vi "PM-A-Acquisition_main_DAQmx.vi"(8 "error in":errorcluster, 11 "init_cluster":T1) -> (0 "error out":errorcluster)   [LabVIEW 2018]
uses:
  init-close/PM-init-data_cluster.ctl
  init-close/PM-init-user_events.ctl
  init-close/PM-common-heartrate_data.ctl
  init-close/PM-common-peak-detect_settings.ctl
  PM-A-aqn_loop_data.ctl
panel:
  in  "Stop":bool
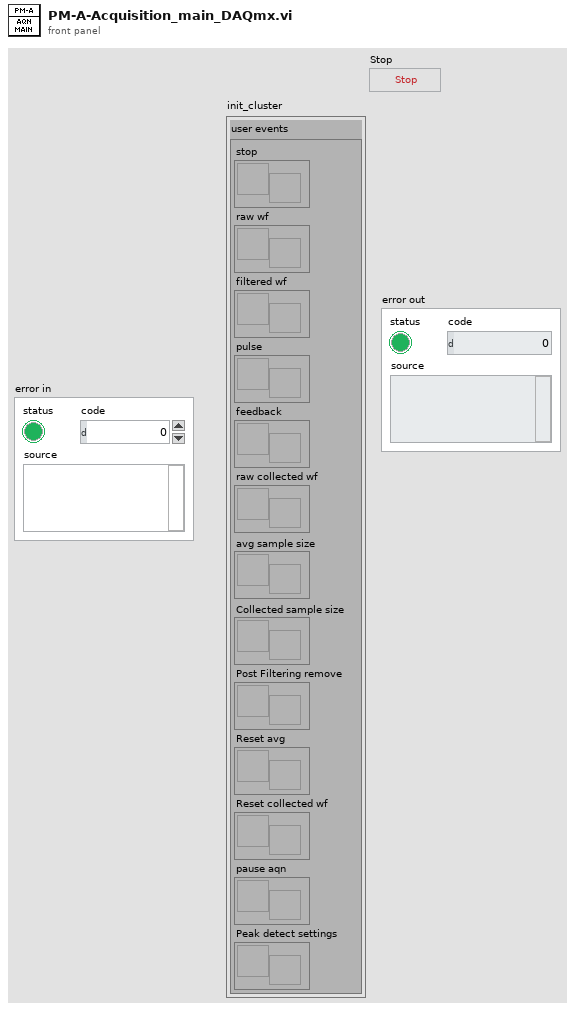
[diagram p1: front panel]
types:
  T1 = typedef "PM-init-data_cluster.ctl" = cluster{"user events":T2}
  T2 = typedef "PM-init-user_events.ctl" = cluster{"stop":refnum<user-event>, "raw wf":refnum<user-event>, "filtered wf":refnum<user-event>, "pulse":refnum<user-event>, "feedback":refnum<user-event>, "raw collected wf":refnum<user-event>, "avg sample size":refnum<user-event>, "Collected sample size":refnum<user-event>, "Post Filtering remove":refnum<user-event>, "Reset avg":refnum<user-event>, "Reset collected wf":refnum<user-event>, "pause aqn":refnum<user-event>, "Peak detect settings":refnum<user-event>}
  T3 = typedef "PM-A-aqn_loop_data.ctl" = cluster{"Stop event":refnum<user-event>, "Raw wf event":refnum<user-event>}
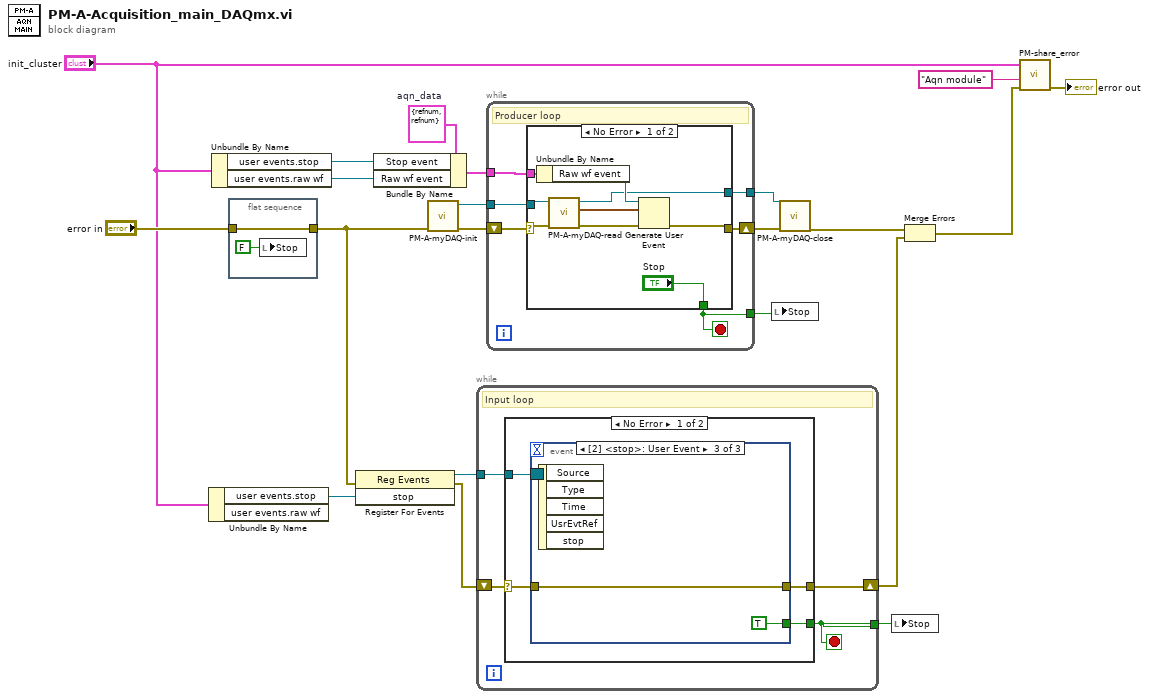
[diagram p0: block diagram]
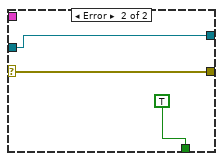
[diagram p2: hidden frame]
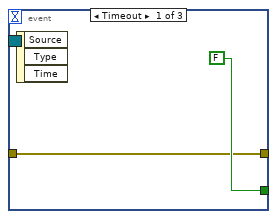
[diagram p3: hidden frame]
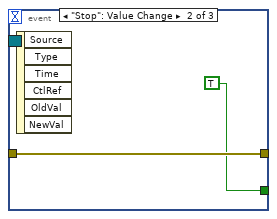
[diagram p4: hidden frame]
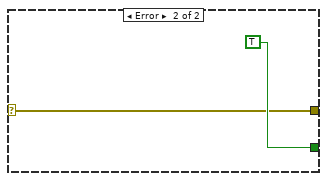
[diagram p5: hidden frame]
diagram:
  w15 = T3 {"Stop event"=refnum, "Raw wf event"=refnum}  # aqn_data
  n1 = Unbundle By Name("init_cluster") -> ("user events.stop"=w17:refnum<user-event>)  [unwired: 1 out]
  n2 = Unbundle By Name("init_cluster") -> ("user events.stop"=w13:refnum<user-event>, "user events.raw wf"=w12:refnum<user-event>)
  n3 = flat-sequence {
    tunnel: "error in" -> [w22]
    tunnel: [w22] -> w6
    frame #0 {
      n4 = local write "Stop"(FALSE ("Stop")) -> ()
    }
  }
  n5 = register-events(error in=w6, w17) -> (reference out=w16:refnum<event-registration>, error out=w18:errorcluster)  [unwired: 1 in]
  n6 = Bundle By Name(cluster=w15, "Stop event"=w13, "Raw wf event"=w12) -> (w14:T3)
  n7 = call "PM-A-myDAQ-init.vi"("error in"=w6) -> ("error out"=w5:errorcluster, "Refnum out"=w4:refnum<k21>)  [unwired: 9 in]
  n8 = while {
    tunnel: [w26] -> w20
    shift-right: [w25] -> w19
    shift-left: w18 -> [w27]
    tunnel: w16 -> [w24]
    stop <- w26 stop-if-true
    # "Input loop"
    n9 = case shown="No Error" w27 {
      selector: w27 -> [w29 w38]
      tunnel: [w31 TRUE] -> w26
      tunnel: [w30 w38] -> w25
      tunnel: w24 -> [w28 _]
      frame No Error {
        n10 = event shown="[2] <stop>: User Event" {
          selector: w28 -> [_ _ _]
          dyn-events: _ -> [_ _ _]
          timeout: _ -> [_ _ _]
          tunnel: [FALSE TRUE TRUE] -> w31
          tunnel: [w32 w35 w37] -> w30
          tunnel: w29 -> [w32 w35 w37]
          event Timeout {
            n11 = event-data() -> ()  [unwired: 1 in, 3 out]
          }
          event "Stop": Value Change {
            n12 = event-data() -> ()  [unwired: 1 in, 6 out]
          }
          event User Event {
            n13 = event-data() -> ()  [unwired: 1 in, 5 out]
          }
        }
      }
      frame Error {
      }
    }
  }
  n14 = while {
    shift-right: [w44] -> w3
    shift-left: w5 -> [w45]
    tunnel: [w43] -> w21
    tunnel: w14 -> [w42]
    tunnel: w4 -> [w41]
    tunnel: [w40] -> w1
    stop <- w43 stop-if-true
    # "Producer loop"
    n15 = case shown="No Error" w45 {
      selector: w45 -> [w50 w57]
      tunnel: ["Stop" TRUE ("Stop")] -> w43
      tunnel: [w47 w57] -> w44
      tunnel: w42 -> [w53 _]
      tunnel: w41 -> [w51 w55]
      tunnel: [w46 w55] -> w40
      frame No Error {
        n16 = Unbundle By Name(w53) -> ("Raw wf event"=w52:refnum<user-event>)
        n17 = call "PM-A-myDAQ-read.vi"("error in (no error)"=w50, "Refnum in"=w51) -> ("error out"=w48:errorcluster, "data"=w49:waveform(dbl), "Refnum out"=w46:refnum<k21>)  [unwired: 7 in]
        n18 = Generate User Event(user event=w52, event data cluster=w49, error in=w48) -> (error out=w47:errorcluster)  [unwired: 1 in, 1 out]
      }
      frame Error {
      }
    }
  }
  n19 = local write "Stop"(w21) -> ()
  n20 = call "PM-A-myDAQ-close.vi"("error in (no error)"=w3, "Refnum in"=w1) -> ("error out"=w2:errorcluster)  [unwired: 9 in]
  n21 = local write "Stop"(w20) -> ()
  n22 = Merge Errors(w2, w19) -> (w10:errorcluster)
  n23 = call "PM-share_error.vi"("error in (no error)"=w10, "module name"="Aqn module", "init_cluster"="init_cluster") -> ("error out"=→"error out":errorcluster)  [unwired: 8 in]
